vi "Convert SmartSyntax to FormatString.vi"(8 "error in (no error)":errorcluster, 11 "Smart Syntax":string) -> (0 "error out":errorcluster, 3 "Scan Syntax Format":T1)   [LabVIEW 2019]
uses:
  Scan Syntax Format.ctl
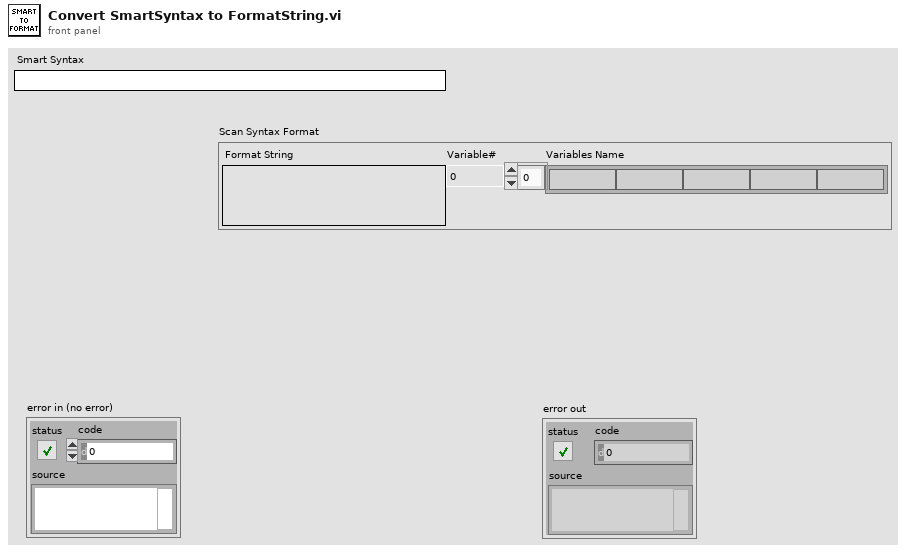
[diagram p1: front panel]
types:
  T1 = typedef "Scan Syntax Format.ctl" = cluster{"Format String":string, "Variable#":i32, "Variables Name":string[]}
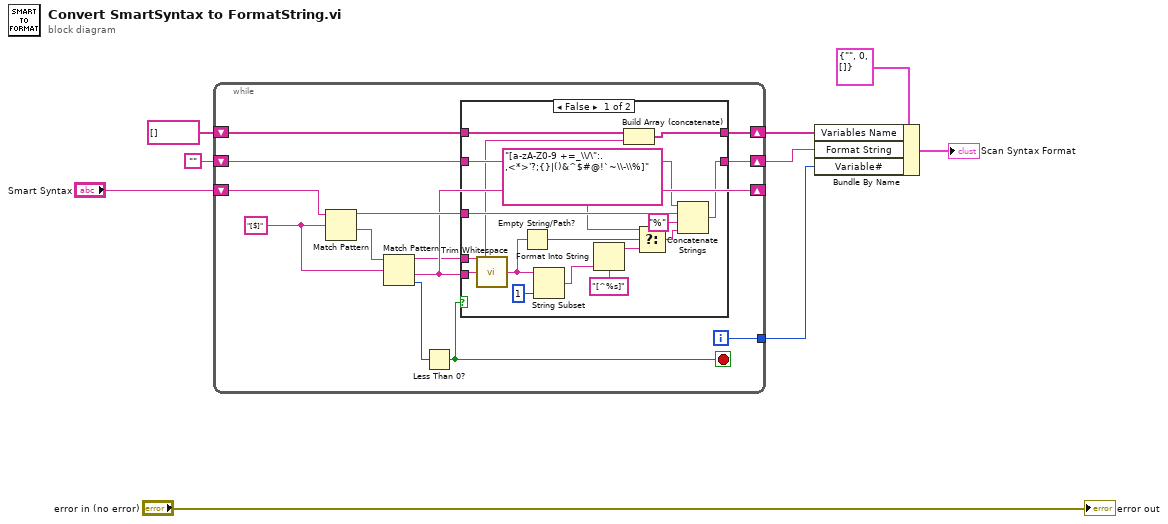
[diagram p0: block diagram]
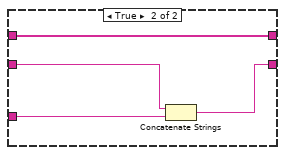
[diagram p2: hidden frame]
diagram:
  n1 = while {
    shift-right: [w14] -> _
    shift-left: "Smart Syntax" -> [w20]
    shift-right: [w16] -> w4
    shift-left: "" -> [w18]
    shift-right: [w12] -> w3
    shift-left: string[] [] ("Variables") -> [w13]
    tunnel: [w10] -> w1
    i -> [w10]
    stop <- w19 stop-if-true
    w22 = "[$]" ("regular expression")
    n2 = Match Pattern(string=w20, regular expression=w22) -> (before substring=w17:string, after substring=w15:string)  [unwired: 1 in, 2 out]
    n3 = Match Pattern(string=w15, regular expression=w22) -> (before substring=w11:string, after substring=w14:string, offset past match=w21:i32)  [unwired: 1 in, 1 out]
    n4 = Less Than 0?(x=w21) -> (x < 0?=w19:bool)
    n5 = case shown="False" w19 {
      tunnel: w18 -> [w37 w41]
      tunnel: w17 -> [w38 w42]
      tunnel: [w36 w40] -> w16
      tunnel: w14 -> [w35 _]
      tunnel: w13 -> [w26 w39]
      tunnel: [w25 w39] -> w12
      tunnel: w11 -> [w24 _]
      frame False {
        n6 = call <vilib>:"Trim Whitespace.vi"("string"=w35) -> ("trimmed string"=w30:string)  [unwired: 1 in]
        n7 = Empty String/Path?(string/path=w30) -> (empty?=w31:bool)
        n8 = String Subset(string=w30, length (rest)=1 ("length (rest)")) -> (substring=w29:string)  [unwired: 1 in]
        n9 = Format Into String(format string="[^%s]", w29) -> (resulting string=w32:string)  [unwired: 2 in, 1 out]
        n10 = Build Array (concatenate)(w26, w24) -> (w25:string[])
        n11 = Select(t="[a-zA-Z0-9 +=_\\/\":.,<*>'?;{}|()&^$#@!`~\\-\\%]" ("format string"), s=w31, f=w32) -> (s? t:f=w27:string)
        n12 = Concatenate Strings(w37, w38, "%" ("string"), w27) -> (w36:string)
      }
      frame True {
        n13 = Concatenate Strings(w41, w42) -> (w40:string)
      }
    }
  }
  n14 = Bundle By Name(cluster=T1 {"Format String"="", "Variable#"=0, "Variables Name"=[]} ("Syntax Format"), "Variables Name"=w3, "Format String"=w4, "Variable#"=w1) -> (→"Scan Syntax Format":T1)
  "error out" <- "error in (no error)"
